vi "Test Google - URL - Build (for stock ticker) - 02.vi"(8 "error in (no error)":errorcluster, 11 "TestCase in":refnum<class "TestCase.lvclass">) -> (0 "error out":errorcluster, 3 "TestCase out":refnum<class "TestCase.lvclass">)   [LabVIEW 2011, in "test.lvclass"]
uses:
  test.lvclass
  <vilib>/addons/_JKI Toolkits/VI Tester/TestCase.llb/TestCase.lvclass
  src/Stock Data Control.ctl
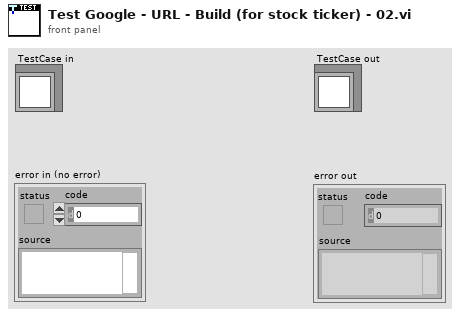
[diagram p1: front panel]
types:
  T1 = typedef "Stock Data Control.ctl" = cluster{"Symbol":string, "Name":string, "Price":string, "Change":string, "Change %":string, "Volume":string}
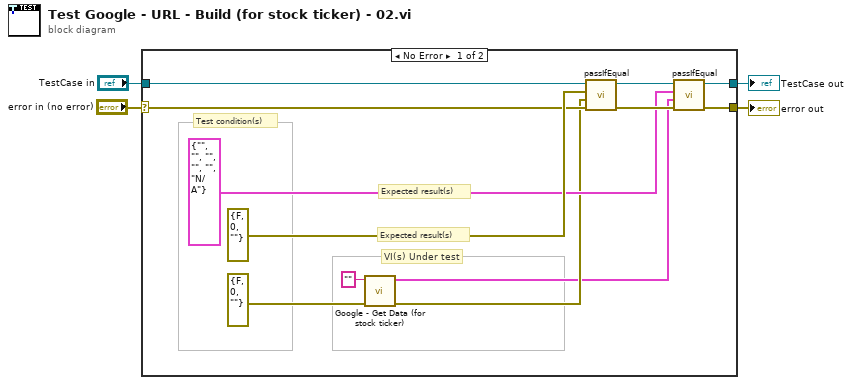
[diagram p0: block diagram]
diagram:
  n1 = case shown="No Error" "error in (no error)" {
    selector: "error in (no error)" -> [w12 w17]
    tunnel: "TestCase in" -> [w13 w18]
    tunnel: [w10 w18] -> w3
    tunnel: [w11 w17] -> w2
    frame No Error {
      # "Expected result(s)"
      # "Expected result(s)"
      # "Test condition(s)"
      # "VI(s) Under test"
      n2 = call "Google - Get Data (for stock ticker).vi"("Symbol"="", "error in"=errorcluster {"status"=FALSE, "code"=0, "source"=""} ("error in (no error)")) -> ("Stock Data"=w5:T1, "error out"=w6:errorcluster)  [unwired: 6 in]
      n3 = call-dynamic "passIfEqual.vi"("error in (no error)"=w12, "y"=w6, "x"=errorcluster {"status"=FALSE, "code"=0, "source"=""} ("error in (no error)"), "TestCase in"=w13) -> ("error out"=w8:errorcluster, "TestCase out"=w9:refnum<class "TestCase.lvclass">)  [unwired: 6 in]
      n4 = call-dynamic "passIfEqual.vi"("error in (no error)"=w8, "y"=w5, "x"=T1 {"Symbol"="", "Name"="", "Price"="", "Change"="", "Change %"="", "Volume"="N/A"} ("Stock Data"), "TestCase in"=w9) -> ("error out"=w11:errorcluster, "TestCase out"=w10:refnum<class "TestCase.lvclass">)  [unwired: 6 in]
    }
    frame Error {
    }
  }
  "TestCase out" <- w3
  "error out" <- w2
